vi "provide_note_book_info.vi"(8 "error in (no error)":errorcluster, 10 "notebook string in":string, 11 "ImagingModeDL090130Frame in":refnum<class "ImagingModeDL090130Frame.lvclass">=refnum) -> (0 "error out":errorcluster, 2 "notebook string out":string, 3 "ImagingModeDL090130Frame out":refnum<class "ImagingModeDL090130Frame.lvclass">)   [LabVIEW 2010, in "ImagingModeDL090130Frame.lvclass"]
uses:
  ImagingModeDL090130Frame.lvclass
  ImagingModeDL090923Scaffold/ImagingModeDL090923Scaffold/ImagingModeDL090923Scaffold.lvclass
  common/classes/ErrorController/ErrorController/class_data.vi
  common/classes/ErrorController/ErrorController/ErrorController.lvclass
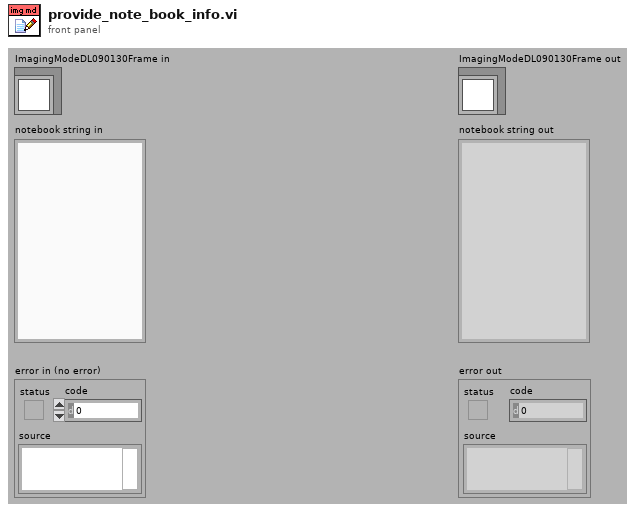
[diagram p1: front panel]
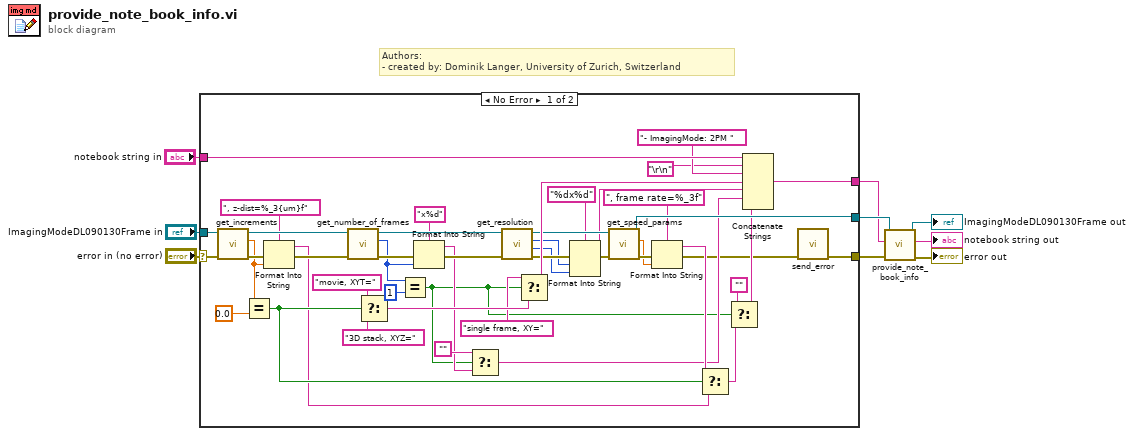
[diagram p0: block diagram]
diagram:
  # "Authors: \n- created by: Dominik Langer, University of Zurich, Switzerland"
  n1 = case shown="No Error" "error in (no error)" {
    selector: "error in (no error)" -> [w53 w58]
    tunnel: "notebook string in" -> [w55 w56]
    tunnel: "ImagingModeDL090130Frame in" -> [w52 w57]
    tunnel: [w11 w58] -> w6
    tunnel: [w42 w57] -> w5
    tunnel: [w19 w56] -> w4
    frame No Error {
      n2 = call-dynamic "get_increments.vi"("error in (no error)"=w53, "ImagingModeDL090130Frame in"=w52) -> ("error out"=w38:errorcluster, "step size"=w18:dbl[unit], "ImagingModeDL090130Frame out"=w51:refnum<class "ImagingModeDL090130Frame.lvclass">)  [unwired: 7 in]
      n3 = Equal?(x=w18, y=dbl[unit] 0.0) -> (x = y?=w39:bool)
      n4 = Format Into String(format string=", z-dist=%_3{um}f", error in=w38, w18) -> (resulting string=w29:string, error out=w37:errorcluster)  [unwired: 1 in]
      n5 = call-dynamic "get_number_of_frames.vi"("error in (no error)"=w37, "ImagingModeDL090130Frame in"=w51) -> ("error out"=w25:errorcluster, "number of frames"=w23:i32, "ImagingModeDL090130Frame out"=w54:refnum<class "ImagingModeDL090130Frame.lvclass">)  [unwired: 7 in]
      n6 = Select(t="movie, XYT=", s=w39, f="3D stack, XYZ=") -> (s? t:f=w46:string)
      n7 = Equal?(x=w23, y=1) -> (x = y?=w16:bool)
      n8 = Format Into String(format string="x%d" ("string"), error in=w25, w23) -> (resulting string=w22:string, error out=w24:errorcluster)  [unwired: 1 in]
      n9 = Select(t="", s=w16, f=w22) -> (s? t:f=w20:string)
      n10 = call-dynamic "get_resolution.vi"("error in (no error)"=w24, "ImagingModeDL090130Frame in"=w54) -> ("error out"=w35:errorcluster, "y resolution"=w32:i32, "x resolution"=w33:i32, "ImagingModeDL090130Frame out"=w43:refnum<class "ImagingModeDL090130Frame.lvclass">)  [unwired: 6 in]
      n11 = Select(t="single frame, XY=", s=w16, f=w46) -> (s? t:f=w44:string)
      n12 = Format Into String(format string="%dx%d", error in=w35, w33, w32) -> (resulting string=w28:string, error out=w34:errorcluster)  [unwired: 1 in]
      n13 = call-dynamic "get_speed_params.vi"("error in (no error)"=w34, "ImagingModeDL090130Frame in"=w43) -> ("error out"=w41:errorcluster, "frame rate"=w40:dbl[unit], "ImagingModeDL090130Frame out"=w42:refnum<class "ImagingModeDL090130Frame.lvclass">)  [unwired: 4 in, 3 out]
      n14 = Format Into String(format string=", frame rate=%_3f", error in=w41, w40) -> (resulting string=w26:string, error out=w12:errorcluster)  [unwired: 1 in]
      n15 = Select(t=w26, s=w39, f=w29) -> (s? t:f=w14:string)
      n16 = Select(t="", s=w16, f=w14) -> (s? t:f=w15:string)
      n17 = Concatenate Strings(w55, "\r\n", "- ImagingMode: 2PM " ("string"), w44, w28, w20, w15) -> (w19:string)
      n18 = call "send_error.vi"("error in (no error)"=w12) -> ("error out"=w11:errorcluster)  [unwired: 10 in]
    }
    frame Error {
    }
  }
  n19 = call-parent "provide_note_book_info.vi"("error in (no error)"=w6, "notebook string in"=w4, "GenericPlugin in"=w5) -> ("error out"=→"error out":errorcluster, "notebook string out"=→"notebook string out":string, "GenericPlugin out"=→"ImagingModeDL090130Frame out":refnum<class "ImagingModeDL090130Frame.lvclass">)  [unwired: 6 in]
